vi "tubo de pitot.vi"(8 "error in (no error)":errorcluster, 10 "noise_gain":dbl, 11 "dimension size":i32) -> (0 "error out":errorcluster, 3 "Array":dbl[](array[numeric]))   [LabVIEW 2019]
panel:
  in  "Tab Control":enum32{"Page 1", "Page 2"}(tab)
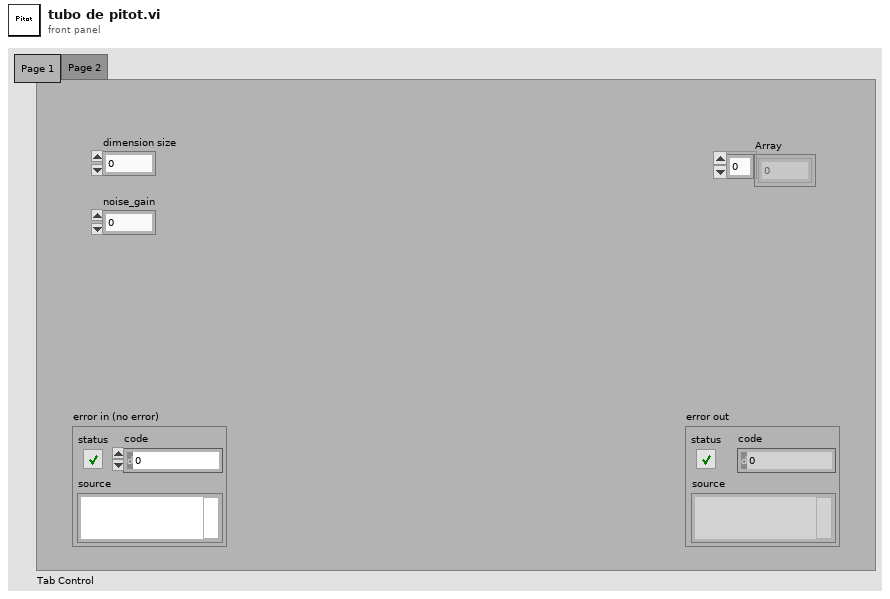
[diagram p1: front panel]
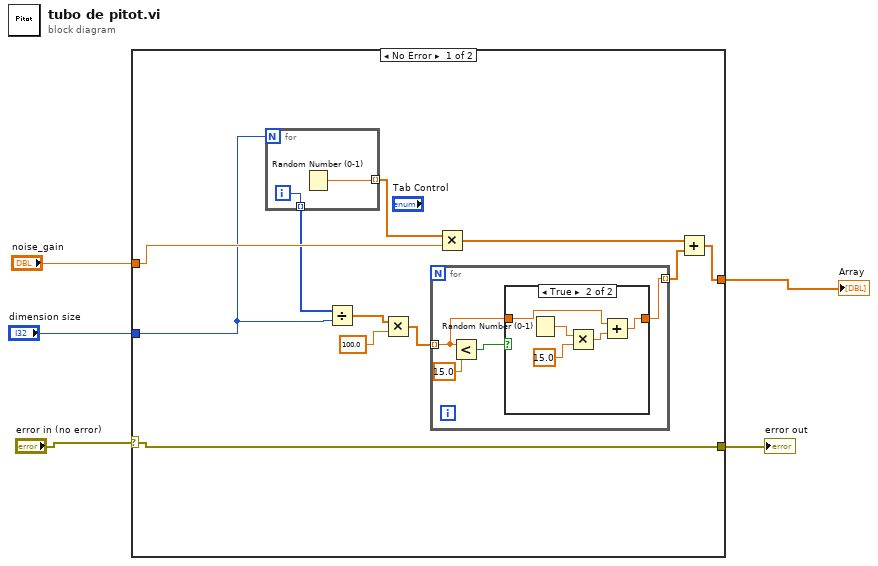
[diagram p0: block diagram]
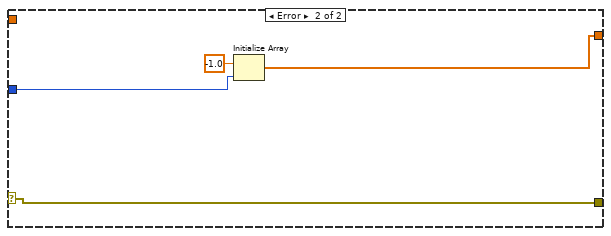
[diagram p3: hidden frame]
diagram:
  n1 = case shown="No Error" "error in (no error)" {
    selector: "error in (no error)" -> [w6 w29]
    tunnel: "dimension size" -> [w11 w32]
    tunnel: "noise_gain" -> [w14 _]
    tunnel: [w6 w29] -> w3
    tunnel: [w13 w30] -> w2
    frame No Error {
      n2 = for {
        N: w11 -> [_]
        tunnel: [w28] -> w16 mode=indexing
        tunnel: [w27] -> w12 mode=indexing
        i -> [w27]
        n3 = Random Number (0-1)() -> (number: 0 to 1=w28:dbl)
      }
      n4 = Divide(x=w12, y=w11) -> (x/y=w10:dbl[])
      n5 = Multiply(x=w10, y=100.0 ("Signal 1")) -> (x*y=w8:dbl[])
      n6 = for {
        tunnel: w8 -> [w18] mode=indexing
        tunnel: [w17] -> w7 mode=indexing
        n7 = Less?(x=w18, y=15.0 ("Signal 1")) -> (x < y?=w19:bool)
        n8 = case shown="True" w19 {
          tunnel: w18 -> [w21 w22]
          tunnel: [w21 w23] -> w17
          frame False {
          }
          frame True {
            n9 = Random Number (0-1)() -> (number: 0 to 1=w26:dbl)
            n10 = Multiply(x=w26, y=15.0) -> (x*y=w24:dbl)
            n11 = Add(x=w22, y=w24) -> (x+y=w23:dbl)
          }
        }
      }
      n12 = Multiply(x=w16, y=w14) -> (x*y=w15:dbl[])
      n13 = Add(x=w15, y=w7) -> (x+y=w13:dbl[])
    }
    frame Error {
      n14 = Initialize Array(-1.0 ("element"), w32) -> (w30:dbl[])
    }
  }
  "error out" <- w3
  "Array" <- w2
